vi "vF.vi"() -> ()   [LabVIEW 2020]
panel:
  out "vF m/s":ext[unit]
  out "x/y":ext[unit]
  in  "vF, eV A":dbl
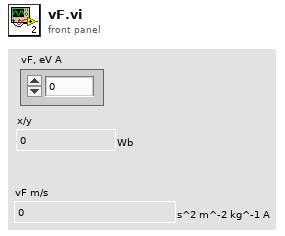
[diagram p1: front panel]
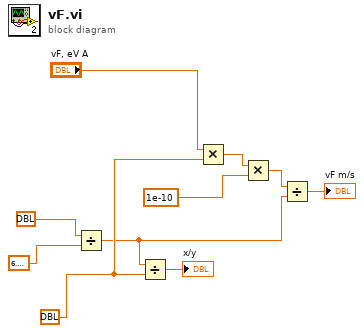
[diagram p0: block diagram]
diagram:
  w6 = ext[unit] 1.6021766208e-19
  n1 = Divide(x=ext[unit] 6.62607004e-34, y=6.283185307179586) -> (x/y=w2:ext[unit])
  n2 = Divide(x=w2, y=w6) -> (x/y=→"x/y":ext[unit])
  n3 = Multiply(x="vF, eV A", y=w6) -> (x*y=w5:ext[unit])
  n4 = Multiply(x=w5, y=1e-10) -> (x*y=w3:ext[unit])
  n5 = Divide(x=w3, y=w2) -> (x/y=→"vF m/s":ext[unit])
